vi "PROJECT CONFIRM STILL ECG.vi"() -> ()   [LabVIEW 2014]
uses:
  <vilib>/MakerHub/LINX/Public/Peripherals/Analog/Analog Read 1 Chan.vi
  <vilib>/MakerHub/LINX/Public/Peripherals/Digital/Digital Write 1 Chan.vi
  <vilib>/MakerHub/LINX/Public/Peripherals/Analog/Analog Read N Chans.vi
  <vilib>/MakerHub/LINX/Public/Peripherals/Digital/Digital Write N Chans.vi
  <vilib>/MakerHub/LINX/Private/Local IO/LinxAnalogRead.vi
  <vilib>/MakerHub/LINX/Public/Utilities/Check Channel.vi
  <vilib>/MakerHub/LINX/Private/Local IO/LinxDigitalWrite.vi
  <vilib>/MakerHub/LINX/Public/Utilities/Open Serial.vi
  <vilib>/MakerHub/LINX/Private/Utilties/Generate Error.vi
  <vilib>/MakerHub/LINX/LMH-LINX.lvlib
panel:
  out "TEMPERATURE":dbl
  out "?":bool
  out "Thermometer":dbl(knob) scale=0.1..100.0
  in  "PORT":refnum<visa-resource-name>
  in  "?":bool
  out "PULSE":bool
  out "ECG":dbl(graph)
  # "ELECTROCARTIOGRAPH"
  # "BODY TEMPERATURE"
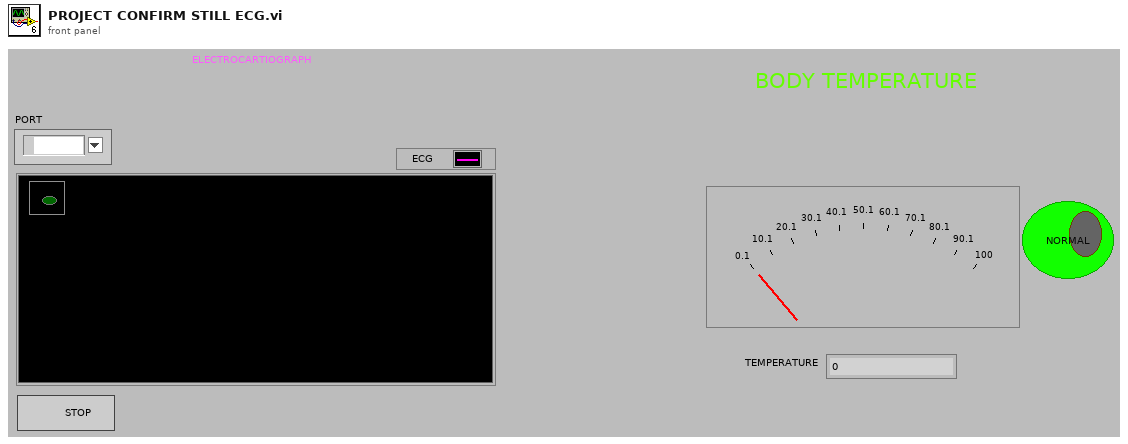
[diagram p1: front panel]
types:
  T1 = typedef "LMH-LINX.lvlib/LINX Ref.ctl" = cluster{"IO":T2, "Interface":T3, "LINX Device Config":T4}
  T2 = typedef "LMH-LINX.lvlib/Platform.ctl" = enum16{"Remote", "Local"}
  T3 = typedef "LMH-LINX.lvlib/Interface.ctl" = enum16{"Serial", "TCP"}
  T4 = typedef "LMH-LINX.lvlib/Device.lvlib/LINX Device Config.ctl" = cluster{"Interface":T3, "COM Port":refnum<visa-resource-name>, "TCP Configuration":T5, "Device Family":u8, "Device ID":u8, "Device Name":string, "TCP Ref":refnum<k5>, "Channels":T6}
  T5 = typedef "LMH-LINX.lvlib/Device.lvlib/TCP Config.ctl" = cluster{"IP Address":string, "Port":u16}
  T6 = typedef "LMH-LINX.lvlib/Channels.ctl" = cluster{"DI":u8[], "DO":u8[], "AI":u8[], "AO":u8[], "PWM":u8[], "QE":u8[], "UART":u8[], "I2C 2":u8[], "SPI":u8[], "CAN":u8[], "Servo":u8[], "AI Ref (V)":dbl, "AI Resolution (Bits)":u8, "AO Ref (V)":dbl, "AO Resolution (Bits)":u8}
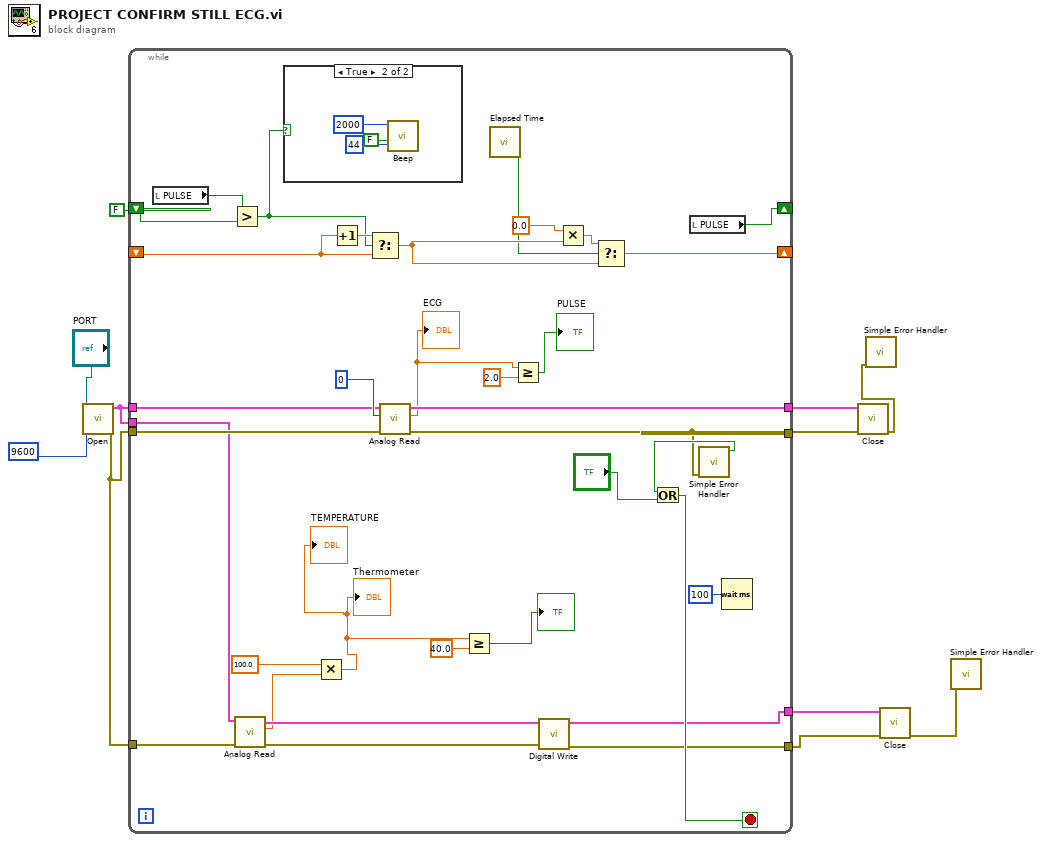
[diagram p0: block diagram]
diagram:
  n1 = call-poly <vilib>:"Open.vi"("Baud Rate Override"=9600 ("code"), "Serial Port"="PORT") -> ("Error Out"=w5:errorcluster, "LINX Resource"=w2:T1)  [unwired: 7 in, 1 out]
  n2 = while {
    tunnel: w5 -> [w45]
    tunnel: [w38] -> w11
    tunnel: w2 -> [w19]
    tunnel: [w42] -> w10
    shift-right: [w29] -> _
    shift-left: _ -> [w33]
    shift-right: [w28] -> _
    shift-left: FALSE -> [w32]
    tunnel: w5 -> [w24]
    tunnel: [w22] -> w4
    tunnel: [w21] -> w3
    tunnel: w2 -> [w12]
    stop <- w40 stop-if-true
    n3 = local read "PULSE"() -> (w31:bool)
    n4 = Greater?(x=w31, y=w32) -> (0:w27:bool)
    n5 = call-poly <vilib>:"Analog Read.vi"("Error In"=w24, "LINX Resource"=w12) -> ("Error Out"=w23:errorcluster, "Voltage"=w18:dbl, "LINX Resource"=w20:T1)  [unwired: 6 in, 1 out]
    n6 = case shown="True" w27 {
      frame False {
      }
      frame True {
        n7 = call <vilib>:"Beep.vi"("use system alert? (T)"=FALSE, "duration (msec)"=u32 44, "frequency (Hz)"=u32 2000) -> ()  [unwired: 9 in]
      }
    }
    n8 = Multiply(x=100.0, y=w18) -> (x*y=w15:dbl)
    "Thermometer" <- w15
    "TEMPERATURE" <- w15
    n9 = Increment(x=w33) -> (x+1=w34:dbl)
    n10 = Select(t=w34, s=w27, f=w33) -> (s? t:f=w36:dbl)
    n11 = call-poly <vilib>:"Analog Read.vi"("Error In"=w45, "Analog Channel"=0, "LINX Resource"=w19) -> ("Error Out"=w38:errorcluster, "Voltage"=w25:dbl, "LINX Resource"=w42:T1)  [unwired: 5 in, 1 out]
    "ECG" <- w25
    n12 = Greater Or Equal?(x=w15, y=40.0) -> (x >= y?=→"?":bool)
    n13 = call "Elapsed Time"() -> ("Time has Elapsed"=w30:bool)  [unwired: 12 in, 7 out]
    n14 = Greater Or Equal?(x=w25, y=2.0) -> (x >= y?=→"PULSE":bool)
    n15 = call-poly <vilib>:"Digital Write.vi"("Error In"=w23, "LINX Resource"=w20) -> ("Error Out"=w22:errorcluster, "LINX Resource"=w21:T1)  [unwired: 8 in]
    n16 = Multiply(x=0.0, y=w36) -> (x*y=w37:dbl)
    n17 = Select(t=w37, s=w30, f=w36) -> (s? t:f=w29:dbl)
    n18 = local read "PULSE"() -> (w28:bool)
    n19 = call <vilib>:"Simple Error Handler.vi"("error in (no error)"=w38) -> ("error?"=w39:bool)  [unwired: 4 in, 4 out]
    n20 = Or(x=w39, y="?") -> (x .or. y?=w40:bool)
    n21 = Wait (ms)(milliseconds to wait=u32 100) -> ()  [unwired: 1 out]
  }
  n22 = call <vilib>:"Close.vi"("Error In"=w11, "LINX Resource"=w10) -> ("Error Out"=w7:errorcluster)  [unwired: 9 in]
  n23 = call <vilib>:"Simple Error Handler.vi"("error in (no error)"=w7) -> ()  [unwired: 4 in, 5 out]
  n24 = call <vilib>:"Close.vi"("Error In"=w4, "LINX Resource"=w3) -> ("Error Out"=w1:errorcluster)  [unwired: 9 in]
  n25 = call <vilib>:"Simple Error Handler.vi"("error in (no error)"=w1) -> ()  [unwired: 4 in, 5 out]
